vi "Teleop.vi"(10 "Match Info":T1={"Autonomous Elapsed Seconds"=0.0, "TeleOp Elapsed Seconds"=0.0, "Disabled Elapsed Seconds"=0.0, "Visited Autonomous"=FALSE, "Visited TeleOp"=FALSE, "Visited Disabled"=FALSE, "Autonomous Settings"={"Autonomous Style"=enum."Independent", "VI Refnum"=refnum}}, 11 "Call Context":T2) -> ()   [LabVIEW 2013]
doc: "This VI is called for each TeleOp packet received from the DS where the robot is not disabled. It is often used to read from the joysticks and update I/O or to update setpoints for timed control loops. It should complete and return within 20 milliseconds or it may miss DS packets."
uses:
  <vilib>/Rock Robotics/WPI/DriverStation/WPI_DriverStationDerivedRobotMode.ctl
  <vilib>/Rock Robotics/WPI/DriverStation/WPI_DriverStationMatch Info.ctl
  <vilib>/Rock Robotics/WPI/Solenoid/WPI_SolenoidValue.ctl
  Robot Global Data.vi
  <vilib>/Rock Robotics/WPI/Solenoid/WPI_SolenoidSetEnum.vi
  <vilib>/Rock Robotics/WPI/RobotDrive/WPI_RobotDriveArcadeDrive_Standard(NoSaturation).vi
  <vilib>/Rock Robotics/WPI/Joystick/WPI_JoystickGetSetRefNum.vi
  <vilib>/Rock Robotics/WPI/RobotDrive/WPI_RobotDriveGetSetRefNum.vi
panel:
  out "Motor Output":dbl
  out "Numeric 1":dbl(slide) scale=0.0..100.0
  out "Boolean 2":bool
  out "Boolean 1":bool
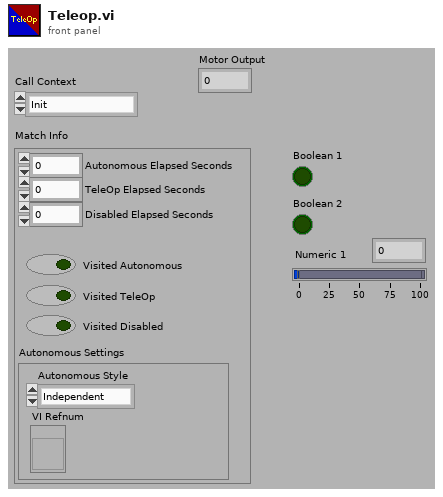
[diagram p1: front panel]
types:
  T1 = typedef "WPI_DriverStationMatch Info.ctl" = cluster{"Autonomous Elapsed Seconds":dbl, "TeleOp Elapsed Seconds":dbl, "Disabled Elapsed Seconds":dbl, "Visited Autonomous":bool, "Visited TeleOp":bool, "Visited Disabled":bool, "Autonomous Settings":cluster{"Autonomous Style":enum16{"Iterative", "Independent"}, "VI Refnum":refnum<vi>}}
  T2 = typedef "WPI_DriverStationDerivedRobotMode.ctl" = enum16{"Init", "Execute", "Stop"}
  T3 = typedef "WPI_SolenoidValue.ctl" = enum16{"Off", "On", "Forward", "Reverse"}
  T4 = typedef "WPI_JoystickDevRef.ctl" = cluster{"Device":T5}
  T5 = typedef "WPI_JoystickDeviceEnum.ctl" = enum16{"USB 1", "USB 2", "USB 3", "USB 4", "Kinect 1", "Kinect 2"}
  T6 = typedef "WPI_JoystickButtonState.ctl" = cluster{"Button 1":bool, "Button 2":bool, "Button 3":bool, "Button 4":bool, "Button 5":bool, "Button 6":bool, "Button 7":bool, "Button 8":bool, "Button 9":bool, "Button 10":bool, "Button 11":bool, "Button 12":bool}
  T7 = cluster{"axis 1 (x)":dbl, "axis 2 (y)":dbl, "axis 3 (throttle)":dbl, "axis 4":dbl, "axis 5":dbl, "axis 6":dbl}
  T8 = typedef "WPI_RobotDriveDevRef.ctl" = cluster{"DevStatus":errorcluster, "Motors[]":T9[], "Square Inputs":bool, "Max Output":dbl, "Isochronous":bool}
  T9 = typedef "WPI_MotorControlDeviceRef.ctl" = cluster{"DeviceStatus":errorcluster, "Type":enum16{"PWM", "CAN"}, "PWM":cluster{"Digital Module":T10, "PWM Channel":T11, "DeadBand":T12}, "CAN":cluster{"Device Number":u8, "Control Mode":T13, "Semaphore":T14, "Max Vout":dbl}, "Invert":bool, "TransformRef":T15, "InvTransformRef":T15}
  T10 = typedef "FPGA_TypedefDigitalModule.ctl" = enum16{"Digital Module 1", "Digital Module 2"}
  T11 = typedef "FPGA_DIOPWMChannel.ctl" = enum8{"PWM 1", "PWM 2", "PWM 3", "PWM 4", "PWM 5", "PWM 6", "PWM 7", "PWM 8", "PWM 9", "PWM 10", "Invalid"}
  T12 = typedef "WPI_PWMDeadband.ctl" = cluster{"Name":string, "maxPositivePwm":i32, "minPositivePwm":i32, "centerPwm":i32, "maxNegativePwm":i32, "minNegativePwm":i32, "angularRange":u16}
  T13 = typedef "WPI_CANJaguar_ControlMode.ctl" = enum8{"Percent VBus", "Current", "Speed", "Position", "Voltage"}
  T14 = typedef "Semaphore RefNum" = refnum<k1>
  T15 = typedef "WPI_PWMTransform_ConPane.ctl" = refnum<vi>
  T16 = typedef "WPI_DigitalInputDevRef.ctl" = cluster{"DevStatus":errorcluster, "DIO Channel":T17, "Digital Module":T10}
  T17 = typedef "FPGA_DIOChannel.ctl" = enum8{"DIO 1", "DIO 2", "DIO 3", "DIO 4", "DIO 5", "DIO 6", "DIO 7", "DIO 8", "DIO 9", "DIO 10", "DIO 11", "DIO 12", "DIO 13", "DIO 14", "Invalid"}
  T18 = typedef "WPI_SolenoidDevRef.ctl" = cluster{"DevStatus":errorcluster, "Solenoid Module":T19, "Forward Solenoid Channel":T20, "Reverse Solenoid Channel":T20}
  T19 = typedef "FPGA_TypedefSolenoidModule.ctl" = enum16{"Solenoid Module 1", "Solenoid Module 2"}
  T20 = typedef "WPI_SolenoidChannel.ctl" = enum8{"Solenoid 1", "Solenoid 2", "Solenoid 3", "Solenoid 4", "Solenoid 5", "Solenoid 6", "Solenoid 7", "Solenoid 8", "Invalid"}
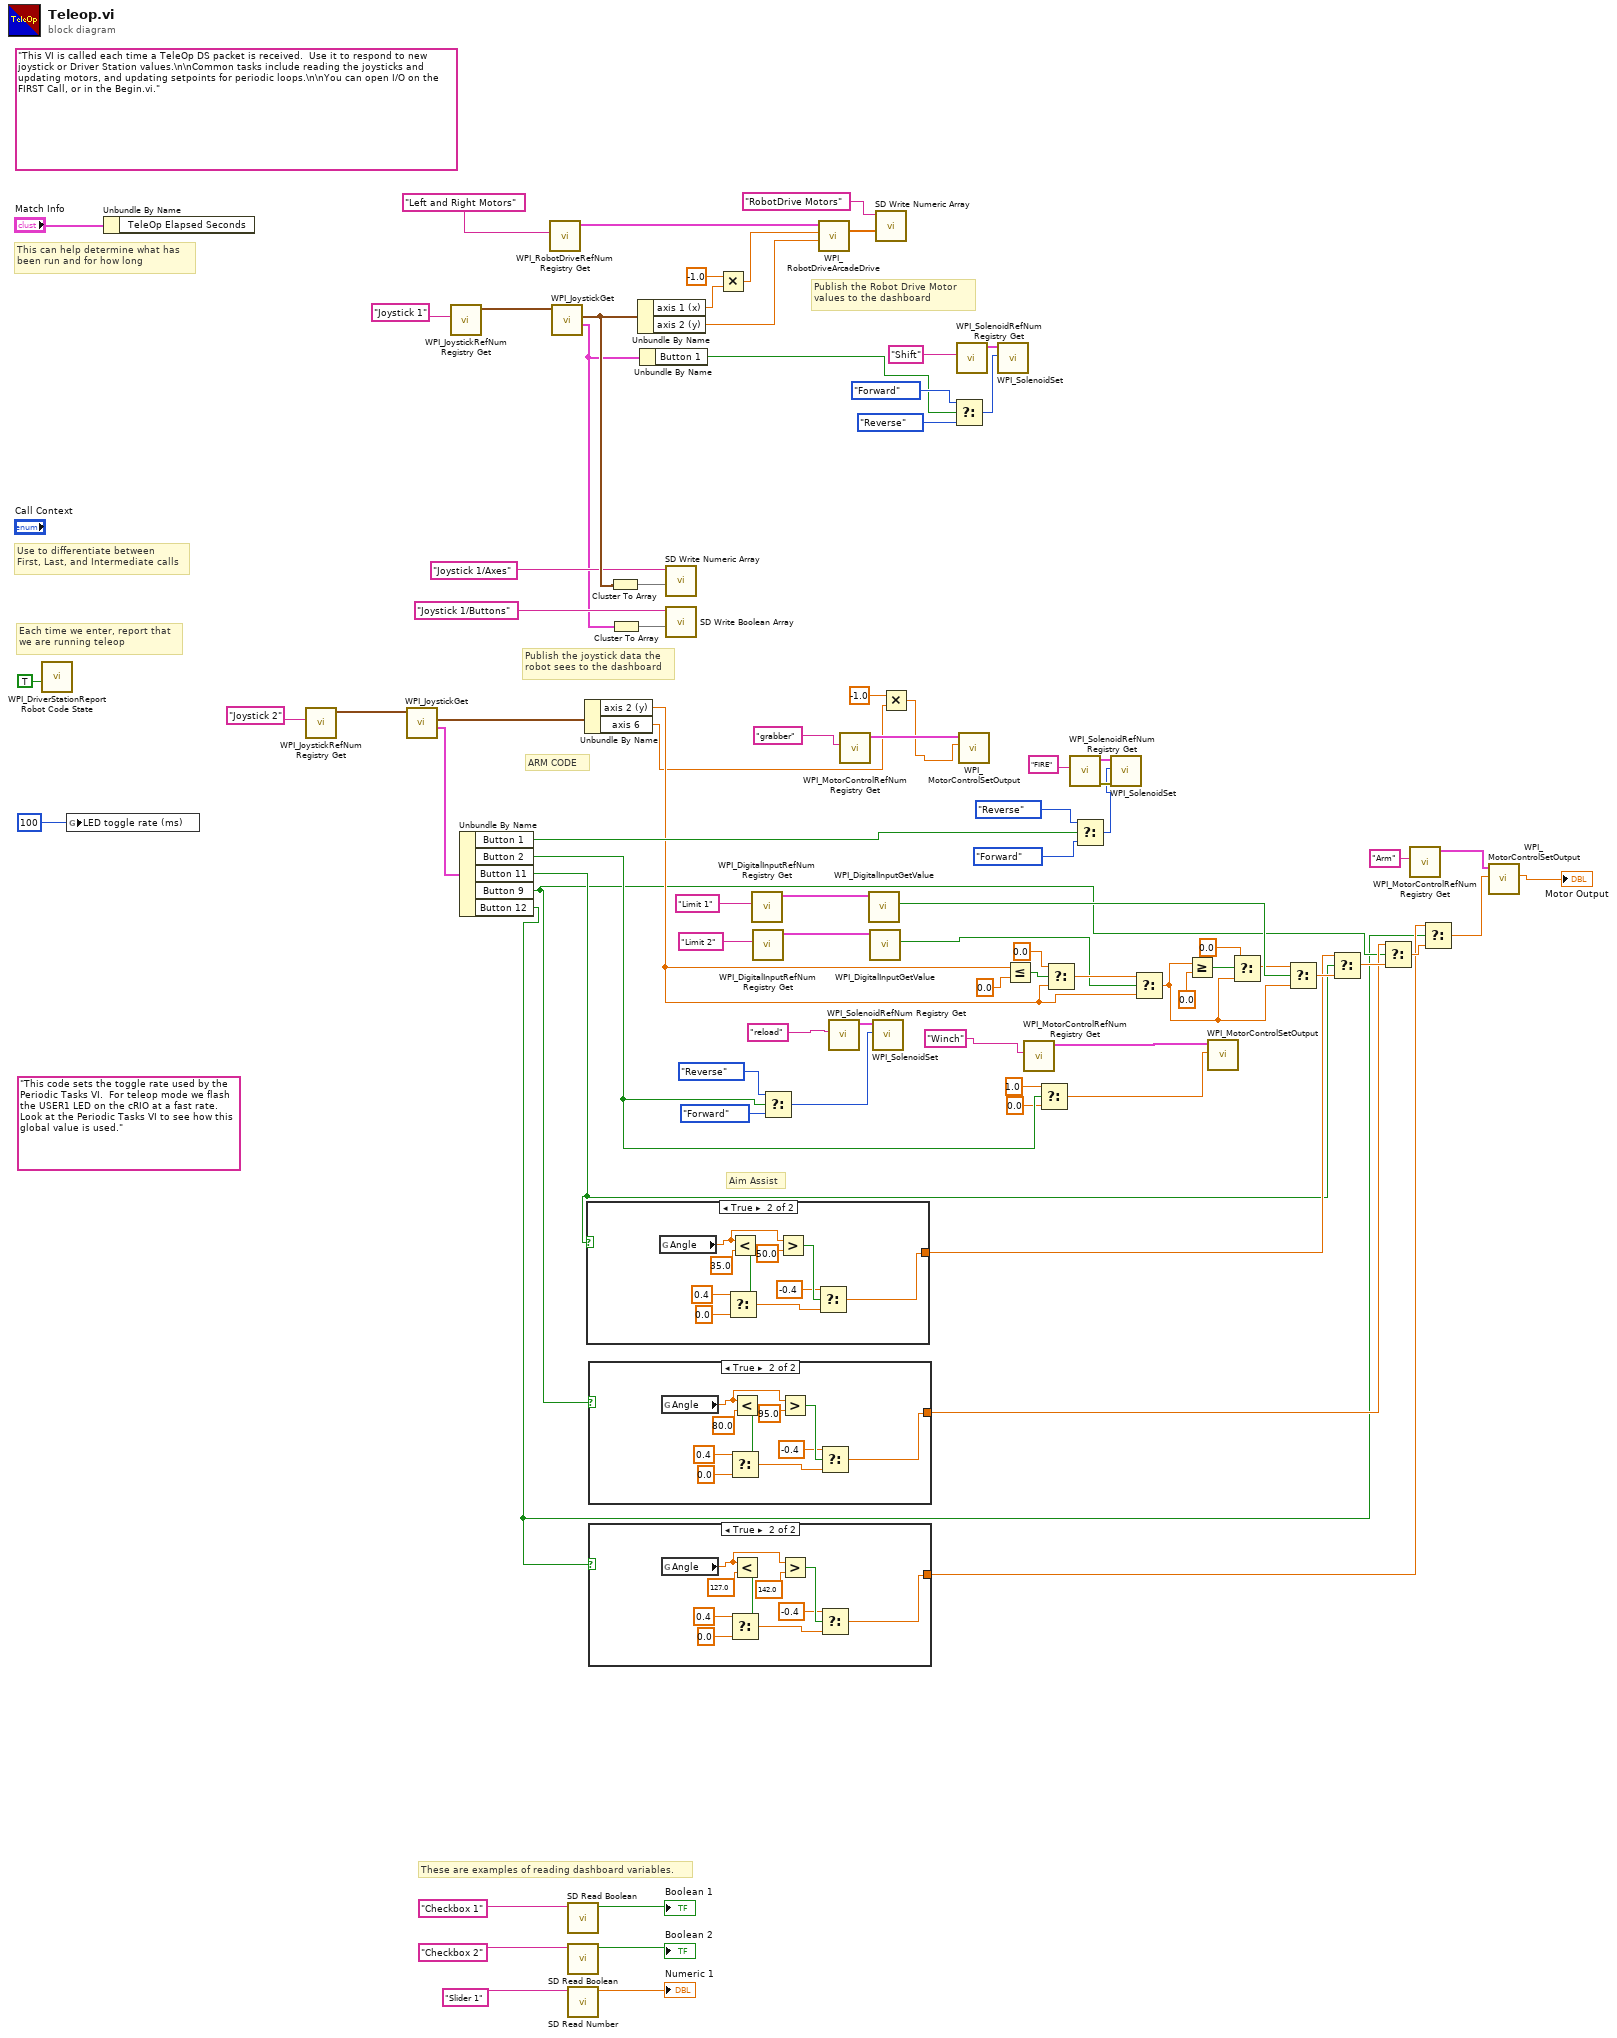
[diagram p0: block diagram]
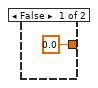
[diagram p2: hidden frame]
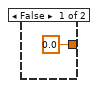
[diagram p3: hidden frame]
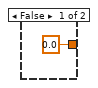
[diagram p4: hidden frame]
diagram:
  (unwired) "This code sets the toggle rate used by the Periodic Tasks VI.  For teleop mode we flash the USER1 LED on the cRIO at a fast rate.  Look at the Periodic Tasks VI to see how this global value is used."
  (unwired) "This VI is called each time a TeleOp DS packet is received.  Use it to respond to new joystick or Driver Station values.\n\nCommon tasks include reading the joysticks and updating motors, and updating setpoints for periodic loops.\n\nYou can open I/O on the FIRST Call, or in the Begin.vi."
  # "Aim Assist"
  # "ARM CODE"
  # "Publish the Robot Drive Motor\nvalues to the dashboard"
  # "These are examples of reading dashboard variables."
  # "Publish the joystick data the\nrobot sees to the dashboard"
  # "Each time we enter, report that\nwe are running teleop"
  # "Use to differentiate between\nFirst, Last, and Intermediate calls"
  # "This can help determine what has\nbeen run and for how long"
  n1 = call <vilib>:"WPI_DriverStationReport Robot Code State.vi"("TeleOp"=TRUE ("Autonomous")) -> ()  [unwired: 10 in, 1 out]
  n2 = global write "Robot Global Data.vi" "LED toggle rate (ms)"(u32 100 ("LED ms toggle rate")) -> ()
  n3 = Unbundle By Name("Match Info") -> ()  [unwired: 1 out]
  n4 = call <vilib>:"WPI_JoystickRefNum Registry Get.vi"("refnum name"="Joystick 2") -> ("JoystickDevRef"=w66:T4)  [unwired: 1 in, 9 out]
  n5 = call <vilib>:"WPI_JoystickGet.vi"("JoystickDevRef"=w66) -> ("Buttons"=w31:T6, "Axes"=w17:T7)  [unwired: 1 in, 4 out]
  n6 = call <vilib>:"WPI_JoystickRefNum Registry Get.vi"("refnum name"="Joystick 1") -> ("JoystickDevRef"=w82:T4)  [unwired: 1 in, 9 out]
  n7 = Unbundle By Name(w31) -> ("Button 1"=w23:bool, "Button 2"=w37:bool, "Button 11"=w14:bool, "Button 9"=w11:bool, "Button 12"=w8:bool)
  n8 = call <vilib>:"WPI_RobotDriveRefNum Registry Get.vi"("refnum name"="Left and Right Motors") -> ("RobotDriveDevRef"=w85:T8)  [unwired: 1 in, 9 out]
  n9 = call <vilib>:"WPI_JoystickGet.vi"("JoystickDevRef"=w82) -> ("Buttons"=w25:T6, "Axes"=w77:T7)  [unwired: 1 in, 4 out]
  n10 = call <vilib>:"SD Read Boolean.vi"("Name"="Checkbox 1" ("refnum name")) -> ("Boolean"=→"Boolean 1":bool)  [unwired: 8 in, 2 out]
  n11 = call <vilib>:"SD Read Boolean.vi"("Name"="Checkbox 2" ("refnum name")) -> ("Boolean"=→"Boolean 2":bool)  [unwired: 8 in, 2 out]
  n12 = call <vilib>:"SD Read Number.vi"("Name"="Slider 1" ("refnum name")) -> ("Numeric"=→"Numeric 1":dbl)  [unwired: 8 in, 2 out]
  n13 = Unbundle By Name(w17) -> ("axis 2 (y)"=w18:dbl, "axis 6"=w3:dbl)
  n14 = case shown="True" w14 {
    tunnel: [0.0 ("f") w89] -> w15
    frame False {
    }
    frame True {
      n15 = global read "Robot Global Data.vi" "Angle"() -> (w94:dbl)
      n16 = Less?(x=w94, y=35.0) -> (x < y?=w97:bool)
      n17 = Select(t=0.4, s=w97, f=0.0) -> (s? t:f=w90:dbl)
      n18 = Greater?(x=w94, y=50.0) -> (0:w92:bool)
      n19 = Select(t=-0.4, s=w92, f=w90) -> (s? t:f=w89:dbl)
    }
  }
  n20 = case shown="True" w11 {
    tunnel: [0.0 ("f") w100] -> w12
    frame False {
    }
    frame True {
      n21 = global read "Robot Global Data.vi" "Angle"() -> (w105:dbl)
      n22 = Less?(x=w105, y=80.0) -> (x < y?=w108:bool)
      n23 = Select(t=0.4, s=w108, f=0.0) -> (s? t:f=w101:dbl)
      n24 = Greater?(x=w105, y=95.0) -> (0:w103:bool)
      n25 = Select(t=-0.4, s=w103, f=w101) -> (s? t:f=w100:dbl)
    }
  }
  n26 = case shown="True" w8 {
    tunnel: [0.0 ("f") w111] -> w9
    frame False {
    }
    frame True {
      n27 = global read "Robot Global Data.vi" "Angle"() -> (w116:dbl)
      n28 = Less?(x=w116, y=127.0) -> (x < y?=w119:bool)
      n29 = Select(t=0.4, s=w119, f=0.0) -> (s? t:f=w112:dbl)
      n30 = Greater?(x=w116, y=142.0) -> (0:w114:bool)
      n31 = Select(t=-0.4, s=w114, f=w112) -> (s? t:f=w111:dbl)
    }
  }
  n32 = Cluster To Array(cluster=w77) -> (array=w76:dbl[])
  n33 = Cluster To Array(cluster=w25) -> (array=w79:bool[])
  n34 = Unbundle By Name(w77) -> ("axis 1 (x)"=w22:dbl, "axis 2 (y)"=w84:dbl)
  n35 = Unbundle By Name(w25) -> ("Button 1"=w24:bool)
  n36 = call <vilib>:"SD Write Numeric Array.vi"("Numeric Array"=w76, "Name"="Joystick 1/Axes") -> ()  [unwired: 8 in, 2 out]
  n37 = call <vilib>:"SD Write Boolean Array.vi"("Boolean Array"=w79, "Name"="Joystick 1/Buttons") -> ()  [unwired: 8 in, 2 out]
  n38 = Multiply(x=-1.0, y=w22) -> (x*y=w20:dbl)
  n39 = call <vilib>:"WPI_DigitalInputRefNum Registry Get.vi"("refnum name"="Limit 1") -> ("DigitalInputDevRef"=w63:T16)  [unwired: 9 in, 1 out]
  n40 = call <vilib>:"WPI_DigitalInputRefNum Registry Get.vi"("refnum name"="Limit 2") -> ("DigitalInputDevRef"=w64:T16)  [unwired: 9 in, 1 out]
  n41 = Select(t=WPI_SolenoidValue."Reverse" ("Value"), s=w37, f=WPI_SolenoidValue."Forward" ("Value")) -> (s? t:f=w40:T3)
  n42 = call-poly <vilib>:"WPI_RobotDriveArcadeDrive.vi"("Y axis value"=w84, "X axis value"=w20, "RobotDriveDevRef"=w85) -> ("Motor Values"=w73:dbl[])  [unwired: 6 in, 2 out]
  n43 = call <vilib>:"WPI_SolenoidRefNum Registry Get.vi"("refnum name"="reload") -> ("SolenoidDevRef"=w29:T18)  [unwired: 9 in, 1 out]
  n44 = call <vilib>:"WPI_MotorControlRefNum Registry Get.vi"("refnum name"="grabber") -> ("MotorControlDevRef"=w61:T9)  [unwired: 9 in, 1 out]
  n45 = call <vilib>:"WPI_DigitalInputGetValue.vi"("DigitalInputDevRef"=w63) -> ("Value"=w62:bool)  [unwired: 8 in, 2 out]
  n46 = call <vilib>:"WPI_DigitalInputGetValue.vi"("DigitalInputDevRef"=w64) -> ("Value"=w19:bool)  [unwired: 8 in, 2 out]
  n47 = call-poly <vilib>:"WPI_SolenoidSet.vi"("Value"=w40, "SolenoidDevRef"=w29) -> ()  [unwired: 8 in, 2 out]
  n48 = call <vilib>:"SD Write Numeric Array.vi"("Numeric Array"=w73, "Name"="RobotDrive Motors") -> ()  [unwired: 8 in, 2 out]
  n49 = Multiply(x=-1.0, y=w3) -> (x*y=w1:dbl)
  n50 = Select(t=WPI_SolenoidValue."Forward" ("Value"), s=w24, f=WPI_SolenoidValue."Reverse" ("Value")) -> (s? t:f=w26:T3)
  n51 = call <vilib>:"WPI_SolenoidRefNum Registry Get.vi"("refnum name"="Shift") -> ("SolenoidDevRef"=w33:T18)  [unwired: 9 in, 1 out]
  n52 = call <vilib>:"WPI_MotorControlSetOutput.vi"("Output"=w1, "MotorControlDevRef"=w61) -> ()  [unwired: 7 in, 3 out]
  n53 = call-poly <vilib>:"WPI_SolenoidSet.vi"("Value"=w26, "SolenoidDevRef"=w33) -> ()  [unwired: 8 in, 2 out]
  n54 = Less Or Equal?(x=w18, y=0.0 ("f")) -> (x <= y?=w50:bool)
  n55 = call <vilib>:"WPI_MotorControlRefNum Registry Get.vi"("refnum name"="Winch") -> ("MotorControlDevRef"=w39:T9)  [unwired: 9 in, 1 out]
  n56 = Select(t=1.0, s=w37, f=0.0) -> (s? t:f=w34:dbl)
  n57 = Select(t=0.0, s=w50, f=w18) -> (s? t:f=w48:dbl)
  n58 = call <vilib>:"WPI_SolenoidRefNum Registry Get.vi"("refnum name"="FIRE") -> ("error out"=w59:errorcluster, "SolenoidDevRef"=w58:T18)  [unwired: 9 in]
  n59 = Select(t=WPI_SolenoidValue."Reverse" ("Value"), s=w23, f=WPI_SolenoidValue."Forward" ("Value")) -> (s? t:f=w54:T3)
  n60 = call-poly <vilib>:"WPI_SolenoidSet.vi"("error in (no error)"=w59, "Value"=w54, "SolenoidDevRef"=w58) -> ()  [unwired: 7 in, 2 out]
  n61 = Select(t=w48, s=w19, f=w18) -> (s? t:f=w43:dbl)
  n62 = Greater Or Equal?(x=w43, y=0.0) -> (x >= y?=w46:bool)
  n63 = call <vilib>:"WPI_MotorControlSetOutput.vi"("Output"=w34, "MotorControlDevRef"=w39) -> ()  [unwired: 7 in, 3 out]
  n64 = Select(t=0.0, s=w46, f=w43) -> (s? t:f=w44:dbl)
  n65 = Select(t=w44, s=w62, f=w43) -> (s? t:f=w16:dbl)
  n66 = Select(t=w15, s=w14, f=w16) -> (s? t:f=w13:dbl)
  n67 = Select(t=w12, s=w11, f=w13) -> (s? t:f=w10:dbl)
  n68 = call <vilib>:"WPI_MotorControlRefNum Registry Get.vi"("refnum name"="Arm") -> ("MotorControlDevRef"=w4:T9)  [unwired: 9 in, 1 out]
  n69 = Select(t=w9, s=w8, f=w10) -> (s? t:f=w5:dbl)
  n70 = call <vilib>:"WPI_MotorControlSetOutput.vi"("Output"=w5, "MotorControlDevRef"=w4) -> ("Motor Output"=→"Motor Output":dbl)  [unwired: 7 in, 2 out]
